vi "Format Control Info Column.vi"(8 "error in (no error)":errorcluster {"code" format="Error %.0f"}, 9 "Column":T4, 10 "Control Info Cluster":T1, 11 "VIDoc Printer - Confluence In":refnum<class "VIDoc Printer - Confluence.lvclass">) -> (0 "error out":errorcluster {"code" format="Error %.0f"}, 1 "Header":string, 2 "Cell Text":string, 3 "VIDoc Printer - Confluence Out":refnum<class "VIDoc Printer - Confluence.lvclass">, 4 "Viable Value?":bool, 5 "Pixel Width":i16=275)   [LabVIEW 2023, in "VIDoc Printer - Confluence.lvlib" / "VIDoc Printer - Confluence.lvclass"]
uses:
  VIDoc Printer - Confluence.lvclass
  Settings/Confluence Printer Settings/Control Info Column.ctl
  Parsing/TypeDefs/Controls Info Cluster.ctl
  <vilib>/picture/picture.llb/imagedata.ctl
  <vilib>/Utility/miscctls.llb/LVKeyTypeDef.ctl
  VIDoc Printer - Confluence.lvclass/VIDoc Printer - Confluence.ctl
  Printer/VIDoc Printer.lvclass
  <userlib>/_PetranWay/LabVIEW Confluence API/Source/PetranWay_Confluence API.lvlib
  Settings/Confluence Printer Settings/VIDoc Settings - Confluence.lvclass
  Parsing/VIDoc Parsing.lvlib
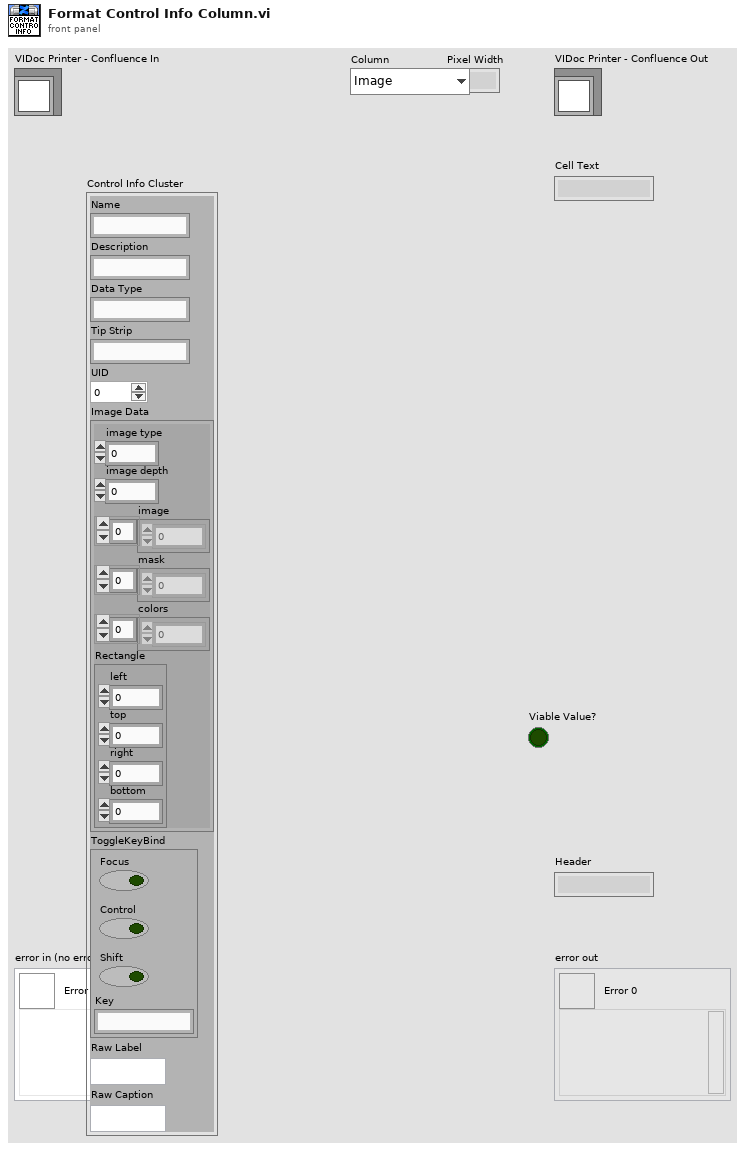
[diagram p1: front panel]
types:
  T1 = typedef "VIDoc Parsing.lvlib/Controls Info Cluster.ctl" = cluster{"Name":string, "Description":string, "Data Type":string, "Tip Strip":string, "UID":i32, "Image Data":T2, "ToggleKeyBind":T3, "Raw Label":string, "Raw Caption":string}
  T2 = typedef "imagedata.ctl" = cluster{"image type":i32, "image depth":i32, "image":u8[], "mask":u8[], "colors":u32[], "Rectangle":cluster{"left":i16, "top":i16, "right":i16, "bottom":i16}}
  T3 = typedef "LVKeyTypeDef.ctl" = cluster{"Focus":bool, "Control":bool, "Shift":bool, "Key":string}
  T4 = typedef "VIDoc Printer - Confluence.lvlib/VIDoc Settings - Confluence.lvclass/Control Info Column.ctl" = enum16{"Image", "Name", "Description", "Caption", "Tip Strip", "Data Type", "Key Toggle"}
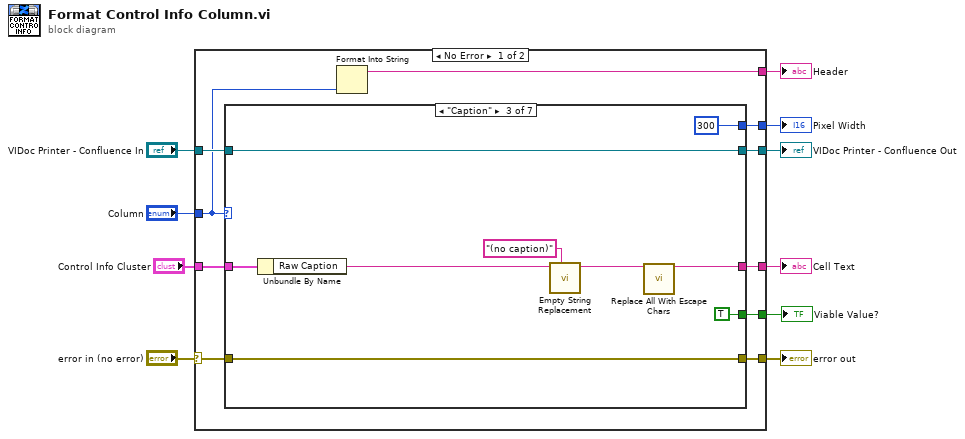
[diagram p0: block diagram]
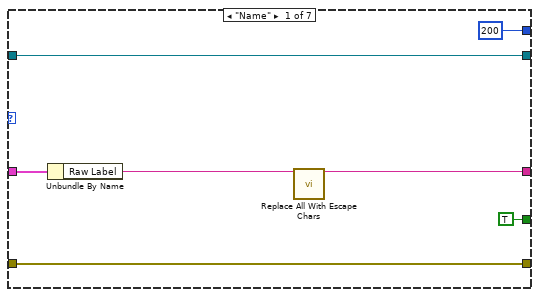
[diagram p2: hidden frame]
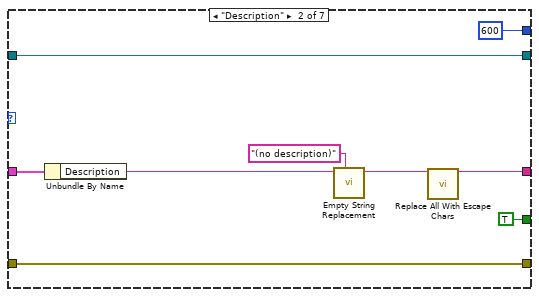
[diagram p3: hidden frame]
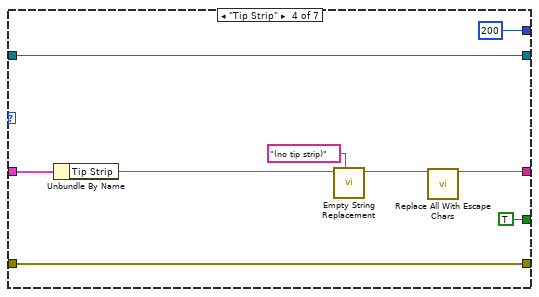
[diagram p4: hidden frame]
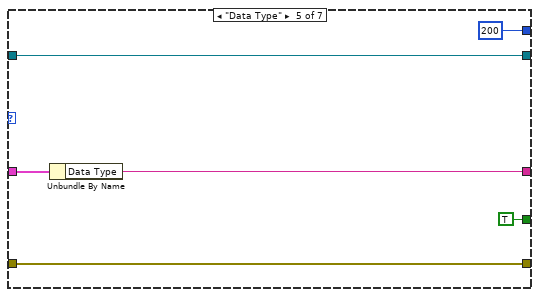
[diagram p5: hidden frame]
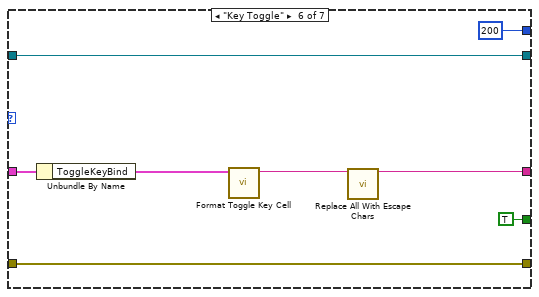
[diagram p6: hidden frame]
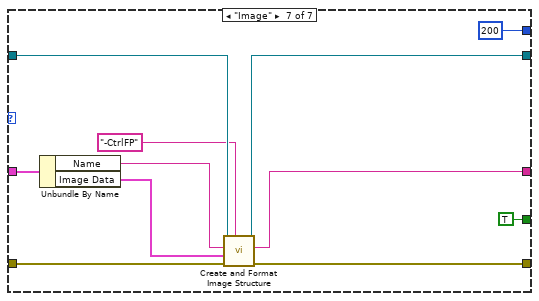
[diagram p7: hidden frame]
diagram:
  n1 = case shown="No Error" "error in (no error)" {
    selector: "error in (no error)" -> [w17 w81]
    tunnel: [w18 w81] -> w9
    tunnel: [w20 w80] -> w7
    tunnel: "VIDoc Printer - Confluence In" -> [w19 w80]
    tunnel: "Column" -> [w16 _]
    tunnel: [w15 _] -> w5
    tunnel: [w14 _] -> w4
    tunnel: "Control Info Cluster" -> [w13 _]
    tunnel: [w12 _] -> w3
    tunnel: [w11 _] -> w2
    frame No Error {
      n2 = case shown="\"Caption\"" w16 {
        tunnel: [w24 w33 w42 w51 w57 w65 w73] -> w20
        tunnel: w19 -> [w24 w33 w42 w51 w57 w65 w74]
        tunnel: [w25 w34 w43 w52 w58 w66 w75] -> w18
        tunnel: w17 -> [w25 w34 w43 w52 w58 w66 w76]
        tunnel: [i16 200 ("Pixel Width") i16 600 ("Pixel Width") i16 300 ("Pixel Width") i16 200 ("Pixel Width") i16 200 ("Pixel Width") i16 200 ("Pixel Width") i16 200 ("Pixel Width")] -> w14
        tunnel: w13 -> [w26 w35 w44 w53 w59 w67 w77]
        tunnel: [w21 w28 w37 w46 w56 w61 w70] -> w12
        tunnel: [TRUE ("File Change Info Available?") TRUE ("File Change Info Available?") TRUE ("File Change Info Available?") TRUE ("File Change Info Available?") TRUE ("File Change Info Available?") TRUE ("File Change Info Available?") TRUE ("File Change Info Available?")] -> w11
        frame "Name" {
          n3 = Unbundle By Name(w26) -> ("Raw Label"=w23:string)
          n4 = call <userlib>:"Replace All With Escape Chars.vi"("Raw String"=w23) -> ("With Substitued Escape Characters"=w21:string)  [unwired: 13 in, 1 out]
        }
        frame "Description" {
          n5 = Unbundle By Name(w35) -> ("Description"=w32:string)
          n6 = call "Empty String Replacement.vi"("Empty"="(no description)", "String"=w32) -> ("String Out"=w29:string)  [unwired: 9 in]
          n7 = call <userlib>:"Replace All With Escape Chars.vi"("Raw String"=w29) -> ("With Substitued Escape Characters"=w28:string)  [unwired: 13 in, 1 out]
        }
        frame "Caption" {
          n8 = Unbundle By Name(w44) -> ("Raw Caption"=w41:string)
          n9 = call "Empty String Replacement.vi"("Empty"="(no caption)", "String"=w41) -> ("String Out"=w38:string)  [unwired: 9 in]
          n10 = call <userlib>:"Replace All With Escape Chars.vi"("Raw String"=w38) -> ("With Substitued Escape Characters"=w37:string)  [unwired: 13 in, 1 out]
        }
        frame "Tip Strip" {
          n11 = Unbundle By Name(w53) -> ("Tip Strip"=w50:string)
          n12 = call "Empty String Replacement.vi"("Empty"="(no tip strip)", "String"=w50) -> ("String Out"=w47:string)  [unwired: 9 in]
          n13 = call <userlib>:"Replace All With Escape Chars.vi"("Raw String"=w47) -> ("With Substitued Escape Characters"=w46:string)  [unwired: 13 in, 1 out]
        }
        frame "Data Type" {
          n14 = Unbundle By Name(w59) -> ("Data Type"=w56:string)
        }
        frame "Key Toggle" {
          n15 = Unbundle By Name(w67) -> ("ToggleKeyBind"=w63:T3)
          n16 = call "Format Toggle Key Cell.vi"("ToggleKeyBind"=w63) -> ("Toggle Key Text"=w62:string)  [unwired: 9 in, 1 out]
          n17 = call <userlib>:"Replace All With Escape Chars.vi"("Raw String"=w62) -> ("With Substitued Escape Characters"=w61:string)  [unwired: 13 in, 1 out]
        }
        frame "Image" {
          n18 = Unbundle By Name(w77) -> ("Name"=w72:string, "Image Data"=w71:T2)
          n19 = call "Create and Format Image Structure.vi"("Name Addition"="-CtrlFP" ("string"), "Error in"=w76, "Image Data"=w71, "Name"=w72, "VIDoc Printer - Confluence In"=w74) -> ("Error out"=w75:errorcluster, "Image Structure Text"=w70:string, "VIDoc Printer - Confluence Out"=w73:refnum<class "VIDoc Printer - Confluence.lvclass">)  [unwired: 3 in, 1 out]
        }
      }
      n20 = Format Into String(w16) -> (resulting string=w15:string)  [unwired: 3 in, 1 out]
    }
    frame Error {
    }
  }
  "error out" <- w9
  "VIDoc Printer - Confluence Out" <- w7
  "Pixel Width" <- w4
  "Cell Text" <- w3
  "Header" <- w5
  "Viable Value?" <- w2
